vi "merFISH_display_scan_new_image.vi"(4 "Display?":bool=TRUE, 5 "error in":errorcluster, 6 "Treated image":T2, 7 "Image contrast":cluster{i32, i32}(slide)={16000, 0} scale=0.0..16000.0, 8 "Real time image":T2) -> (0 "error out":errorcluster, 2 "intensity range":T1, 3 "Image Dst Out":T2)   [LabVIEW 2015]
uses:
  <vilib>/vision/Image Controls.llb/IMAQ Image.ctl
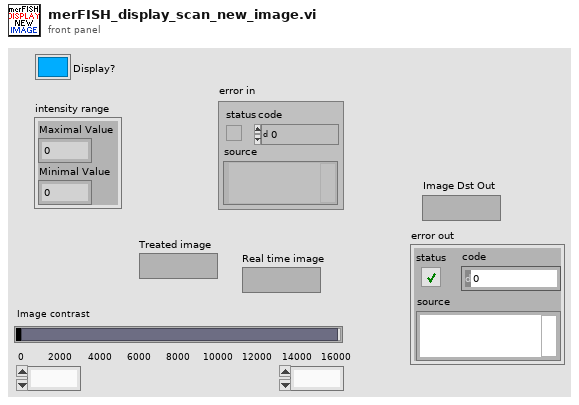
[diagram p1: front panel]
types:
  T1 = cluster{"Maximal Value":sgl, "Minimal Value":sgl}
  T2 = typedef "IMAQ Image.ctl" = refnum<image>
  T3 = cluster{"Mean Value":sgl, "Standard Variation":sgl, "Minimal Value":sgl, "Maximal Value":sgl, "Area (calibrated)":sgl, "Area (pixels)":u32, "%":sgl, "Calibration Valid":bool}
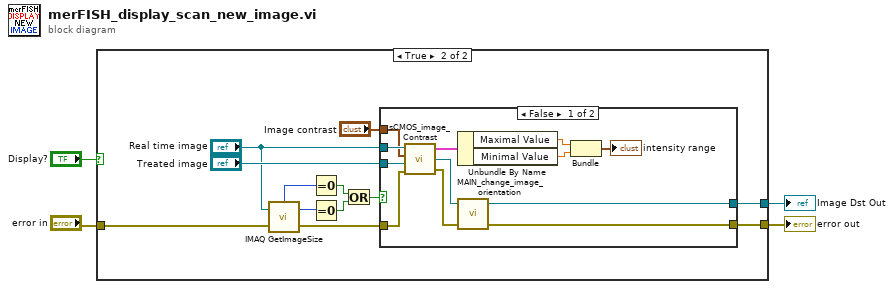
[diagram p0: block diagram]
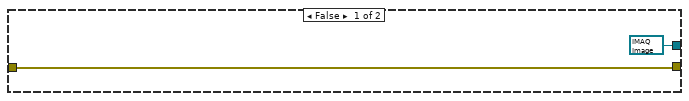
[diagram p2: hidden frame]
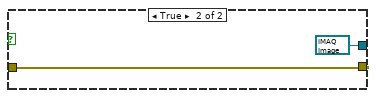
[diagram p3: hidden frame]
diagram:
  n1 = case shown="True" "Display?" {
    tunnel: "error in" -> [w6 w9]
    tunnel: [w6 w8] -> w3
    tunnel: [T2 refnum ("Image Out") w7] -> w1
    frame False {
    }
    frame True {
      n2 = call "IMAQ GetImageSize"("Image"="Real time image", "error in (no error)"=w9) -> ("Y Resolution"=w15:i32, "X Resolution"=w16:i32, "error out"=w11:errorcluster)  [unwired: 2 in]
      n3 = Equal To 0?(x=w16) -> (x = 0?=w14:bool)
      n4 = Equal To 0?(x=w15) -> (x = 0?=w13:bool)
      n5 = Or(x=w14, y=w13) -> (x .or. y?=w12:bool)
      n6 = case shown="False" w12 {
        tunnel: "Treated image" -> [w27 _]
        tunnel: [w20 w32] -> w8
        tunnel: "Real time image" -> [w26 _]
        tunnel: w11 -> [w25 w32]
        tunnel: "Image contrast" -> [w24 _]
        tunnel: [w19 T2 refnum ("Image Out")] -> w7
        frame False {
          n7 = call "sCMOS_image_Contrast.vi"("error in"=w25, "Image Dst"=w27, "Image contrast"=w24, "New Image"=w26) -> ("error out"=w21:errorcluster, "Image Dst Out"=w22:T2, "Global Report"=w30:T3)
          n8 = Unbundle By Name(w30) -> ("Maximal Value"=w29:sgl, "Minimal Value"=w28:sgl)
          n9 = call "MAIN_change_image_orientation.vi"("error in"=w21, "Image IN"=w22) -> ("error out"=w20:errorcluster, "Image Out"=w19:T2)  [unwired: 2 in]
          n10 = Bundle("Maximal Value"=w29, "Minimal Value"=w28) -> (→"intensity range":T1)  [unwired: 1 in]
        }
        frame True {
        }
      }
    }
  }
  "error out" <- w3
  "Image Dst Out" <- w1
